vi "Remove Named Service.vi"(8 "error in (no error)":errorcluster, 10 "Service Name":string, 11 "Service Config Display in":refnum<class "Service Config Display.lvclass">) -> (0 "error out":errorcluster, 3 "Service Config Display out":refnum<class "Service Config Display.lvclass">)   [LabVIEW 2016, in "Assert Display.lvlib" / "Service Config Display.lvlib" / "Service Config Display.lvclass"]
doc: "Removes a named service from the list of active services"
uses:
  Service Config Display.lvclass
  Service Config Display.lvclass/Service Config Display.ctl
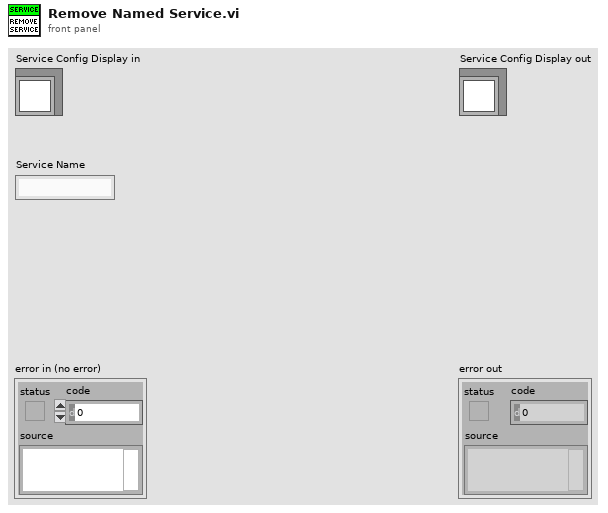
[diagram p1: front panel]
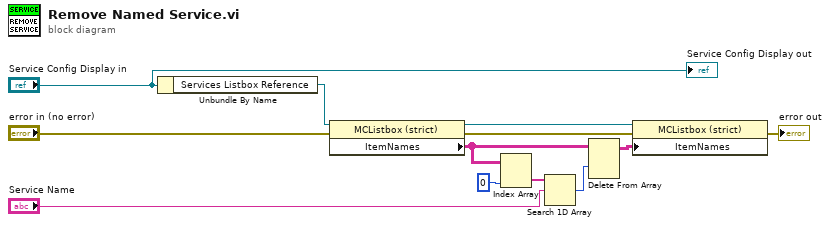
[diagram p0: block diagram]
diagram:
  n1 = Unbundle By Name("Service Config Display in") -> ("Services Listbox Reference"=w8:refnum<vi>)
  n2 = property class="MCListbox (strict)"(reference=w8, error in="error in (no error)") -> (reference out=w3:refnum<vi>, error out=w2:errorcluster, "ItemNames"=w5:string[][])
  n3 = Index Array(array=w5, index (col)=0 ("disabled index (col)")) -> (element=w6:string[])  [unwired: 1 in]
  n4 = Search 1D Array(1D array=w6, element="Service Name") -> (index of element=w4:i32)  [unwired: 1 in]
  n5 = Delete From Array(array=w5, index (row)=w4) -> (array with subset deleted=w1:string[][])  [unwired: 2 in, 1 out]
  n6 = property class="MCListbox (strict)"(reference=w3, error in=w2, "ItemNames"=w1) -> (error out=→"error out":errorcluster)  [unwired: 1 out]
  "Service Config Display out" <- "Service Config Display in"
